vi "String To Timestamp.vi"(8 "error in (no error)":errorcluster, 10 "String":string, 11 "Registry Object":refnum<class "Carya Config.lvclass">) -> (0 "error out":errorcluster, 2 "Unescaped string":timestamp, 3 "Registry Object":refnum<class "Carya Config.lvclass">)   [LabVIEW 2013, in "Carya Config.lvclass"]
doc: "Copyright 2018, Carya Automatisering, Wiebe Walstra."
uses:
  Carya Config.lvclass
  <vilib>/Utility/miscctls.llb/LVDateTimeRec.ctl
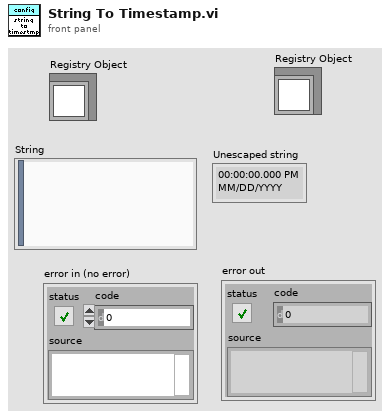
[diagram p1: front panel]
types:
  T1 = typedef "LVDateTimeRec.ctl" = cluster{"fractional second":dbl, "second":i32, "minute":i32, "hour":i32, "day of month":i32, "month":i32, "year":i32, "day of week":i32, "day of year":i32, "DST":i32}
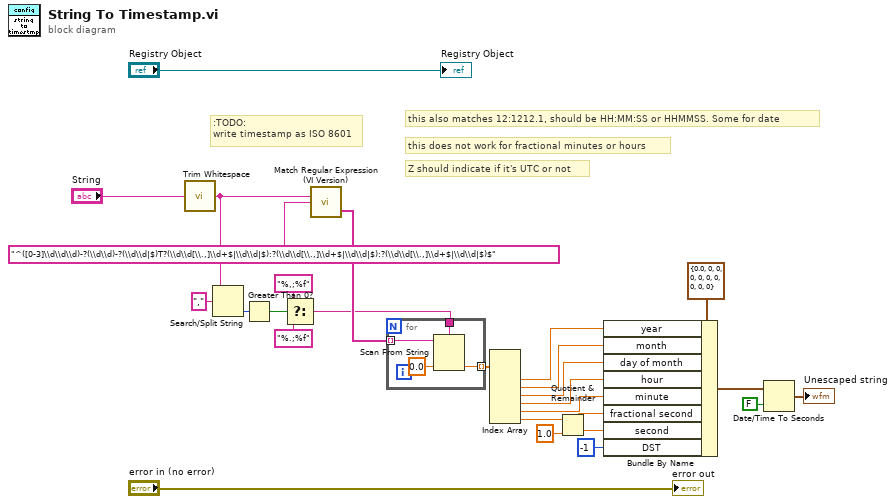
[diagram p0: block diagram]
diagram:
  # "Z should indicate if it's UTC or not"
  # "this does not work for fractional minutes or hours"
  # "this also matches 12:1212.1, should be HH:MM:SS or HHMMSS. Some for date"
  # ":TODO:\nwrite timestamp as ISO 8601"
  n1 = call <vilib>:"Trim Whitespace.vi"("string"="String") -> ("trimmed string"=w23:string)  [unwired: 1 in]
  n2 = Search/Split String(string=w23, search string/char (-)=",") -> (offset of match=w20:i32)  [unwired: 1 in, 2 out]
  n3 = Greater Than 0?(x=w20) -> (x > 0?=w19:bool)
  n4 = Select(t="%,;%f" ("search string/char (-)"), s=w19, f="%.;%f" ("search string/char (-)")) -> (s? t:f=w16:string)
  n5 = call "Match Regular Expression (VI Version).vi"("input string"=w23, "regular expression"="^([0-3]\\d\\d\\d)-?(\\d\\d)-?(\\d\\d|$)T?(\\d\\d[\\.,]\\d+$|\\d\\d|$):?(\\d\\d[\\.,]\\d+$|\\d\\d|$):?(\\d\\d[\\.,]\\d+$|\\d\\d|$)$") -> ("Capturing goups"=w21:string[])  [unwired: 7 in, 6 out]
  n6 = for {
    tunnel: w21 -> [w31] mode=indexing
    tunnel: w16 -> [w30]
    tunnel: [w28] -> w15 mode=indexing
    n7 = Scan From String(format string=w30, input string=w31, default 1=0.0 ("default value 1")) -> (output 1=w28:dbl)  [unwired: 2 in, 3 out]
  }
  n8 = Index Array(array=w15) -> (element #2=w5:dbl, element #3=w6:dbl, element #4=w7:dbl, element #5=w8:dbl, element #6=w9:dbl, element #7=w12:dbl)  [unwired: 7 in, 1 out]
  n9 = Quotient & Remainder(x=w12, y=1.0) -> (x-y*floor(x/y)=w10:dbl, floor(x/y)=w13:dbl)
  n10 = Bundle By Name(cluster=T1 {"fractional second"=0.0, "second"=0, "minute"=0, "hour"=0, "day of month"=0, "month"=0, "year"=0, "day of week"=0, "day of year"=0, "DST"=0} ("date time rec"), "year"=w5, "month"=w6, "day of month"=w7, "hour"=w8, "minute"=w9, "fractional second"=w10, "second"=w13, "DST"=-1) -> (w4:T1)
  n11 = Date/Time To Seconds(1:FALSE ("is UTC (F)"), 2:w4) -> (0:→"Unescaped string":timestamp)
  "Registry Object" <- "Registry Object"
  "error out" <- "error in (no error)"
